vi "DG535 Receive Message.vi"(2 "timeout ms":u32=4294967295 format="%.0x", 3 "address string":string, 4 "byte count":i32, 7 "source":string, 8 "read mode":i32(ring) items=["terminate read on EOI or byte count", "terminate read on EOI, byte count, or CR", "terminate read on EOI, byte count, or LF"], 9 "error in":errorcluster) -> (0 "read buffer":string, 5 "status":bool[](array[boolean]), 6 "error out":errorcluster)   [LabVIEW 2013]
doc: "Sends a string to a message based VXI instrument. In order to communicate with an instrument, you must first open the instrument by running the Open VXI Instrument or running the initialize VI (initialize VIs call the Open VXI Instrument in their block diagram). Use the instrument ID generated by the Open VXI Instrument to address the specific instrument, then set the write mode and enter the string to send. If a write error occurs, error code 1230 is returned. If you fail to open the instrument, error code 1232 is returned."
panel:
  in  "[empty array]":bool[](array[boolean])
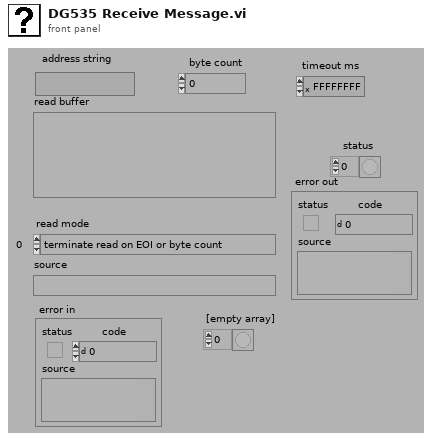
[diagram p1: front panel]
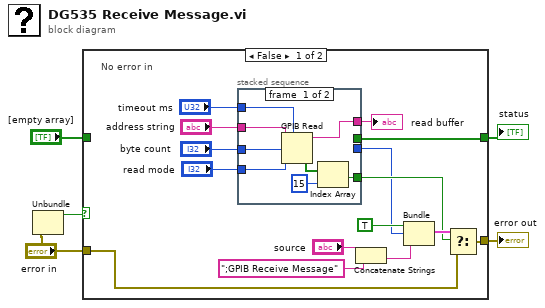
[diagram p0: block diagram]
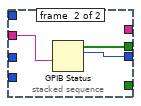
[diagram p2: hidden frame]
diagram:
  n1 = Unbundle("error in") -> ("status"=w1:bool)  [unwired: 2 out]
  n2 = case shown="False" w1 {
    tunnel: "[empty array]" -> [_ w32]
    tunnel: [w16 w32] -> w3
    tunnel: [w19 w33] -> w4
    tunnel: "error in" -> [w10 w33]
    frame False {
      # "No error in"
      n3 = stacked-sequence {
        tunnel: [_ w31] -> w16
        tunnel: [w26 _] -> w17
        tunnel: [_ w30] -> w15
        tunnel: "address string" -> [w25 w29]
        tunnel: "timeout ms" -> [w24 _]
        tunnel: "read mode" -> [w23 _]
        tunnel: "byte count" -> [w22 _]
        tunnel: [w21 _] -> w6
        frame #0 {
          n4 = GPIB Read(0:w25, 1:w22, 2:w23, 4:w24) -> (5:w21:string, 6:w27:bool[])  [unwired: 1 in, 1 out]
          n5 = Index Array(array=w27, index=15) -> (element=w26:bool)
        }
        frame #1 {
          n6 = GPIB Status(0:w29) -> (2:w31:bool[], 3:w30:i16)  [unwired: 1 in, 2 out]
        }
      }
      "read buffer" <- w6
      n7 = Concatenate Strings("source", ";GPIB Receive Message") -> (w11:string)
      n8 = Bundle(TRUE, "GPIB error"=w15, w11) -> (w20:cluster{bool, "GPIB error":i16, string})  [unwired: 1 in]
      n9 = Select(t=w20, s=w17, f=w10) -> (s? t:f=w19:errorcluster)
    }
    frame True {
      # "Error in"
    }
  }
  "status" <- w3
  "error out" <- w4
